vi "value change.vi"(0 "NewVal":string[][](array[string]), 8 "OldVal":string[][](array[string]), 11 "disabled index (col)":i32) -> (3 "x > y?":bool)   [LabVIEW 2015]
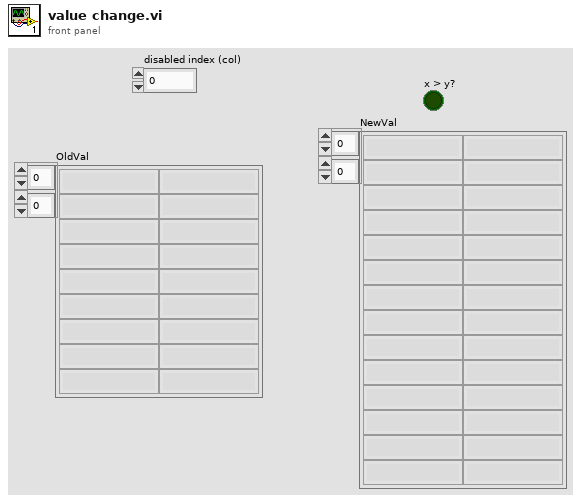
[diagram p1: front panel]
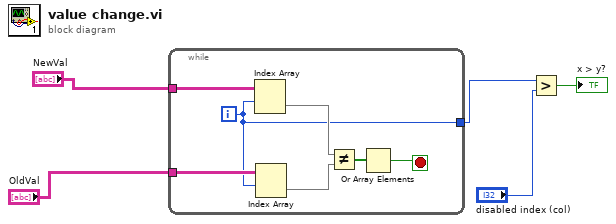
[diagram p0: block diagram]
diagram:
  n1 = while {
    tunnel: "NewVal" -> [w12]
    tunnel: "OldVal" -> [w11]
    tunnel: [w6] -> w3
    i -> [w6]
    stop <- w7 stop-if-true
    n2 = Index Array(array=w12, index (row)=w6) -> (element=w10:string[])  [unwired: 1 in]
    n3 = Index Array(array=w11, index (row)=w6) -> (element=w9:string[])  [unwired: 1 in]
    n4 = Not Equal?(x=w10, y=w9) -> (x != y?=w8:bool[])
    n5 = Or Array Elements(Boolean array=w8) -> (logical OR=w7:bool)
  }
  n6 = Greater?(x=w3, y="disabled index (col)") -> (0:→"x > y?":bool)
